vi "Get Compiler Level.vi"(8 "error in (no error)":errorcluster, 11 "NI_AB_API_EXE in":refnum<class "NI_AB_API_EXE.lvclass">) -> (0 "error out":errorcluster, 2 "compiler Level":u32=1, 3 "NI_AB_API_EXE out":refnum<class "NI_AB_API_EXE.lvclass">)   [LabVIEW 2020, in "NI_AB_API_EXE.lvclass"]
uses:
  <vilib>/AppBuilder/AB_API/EXE/NI_AB_API_EXE.lvclass
  <vilib>/AppBuilder/AB_API/EXE/NI_AB_API_EXE.lvclass/NI_AB_API_EXE.ctl
  <vilib>/AppBuilder/AB_API/Application/NI_AB_API_Application.lvclass
panel:
  # "0: SSE2 optimization disabled\n1: SSE2 optimization enabled"
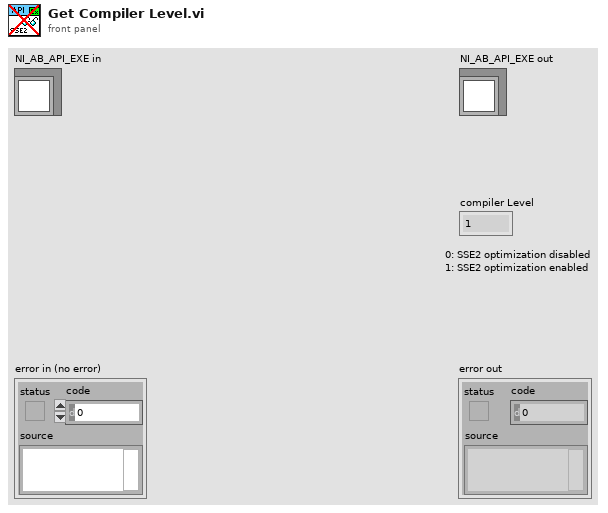
[diagram p1: front panel]
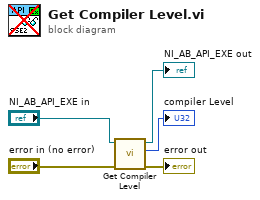
[diagram p0: block diagram]
diagram:
  n1 = call-parent "Get Compiler Level.vi"("error in (no error)"="error in (no error)", "NI_AB_API_Build in"="NI_AB_API_EXE in") -> ("error out"=→"error out":errorcluster, "compiler Level"=→"compiler Level":u32, "NI_AB_API_Build out"=→"NI_AB_API_EXE out":refnum<class "NI_AB_API_EXE.lvclass">)  [unwired: 7 in]
